vi "unmarshalling.vi"(7 "Type":variant, 8 "error in (no error)":errorcluster, 10 "String":string, 11 "Serializer in":refnum<class "Serializer.JKI-JSON.lvclass">) -> (0 "error out":errorcluster, 2 "Variant":variant, 3 "Serializer out":refnum<class "Serializer.JKI-JSON.lvclass">)   [LabVIEW 2017, in "Serializer.JKI-JSON.lvclass"]
uses:
  Serializer.JKI-JSON.lvclass
  <vilib>/addons/_JKI.lib/Serialization/JSON/JKI JSON Serialization.lvlib
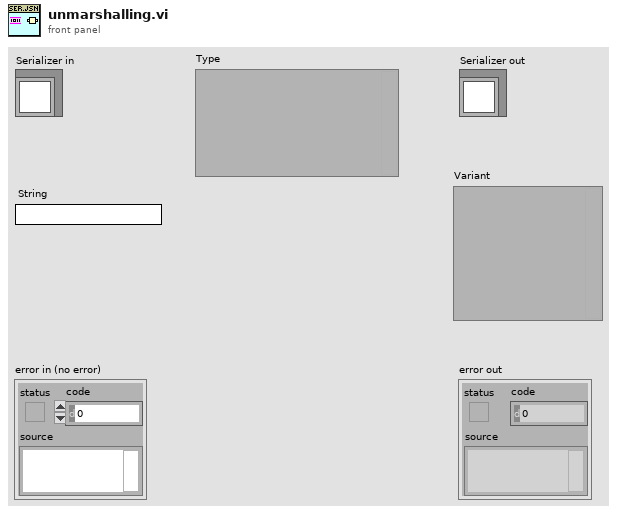
[diagram p1: front panel]
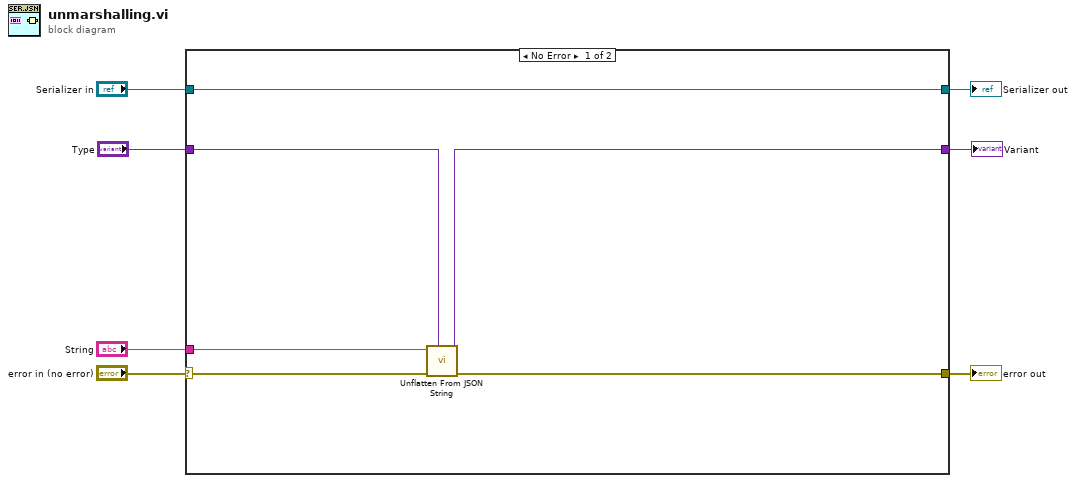
[diagram p0: block diagram]
diagram:
  n1 = case shown="No Error" "error in (no error)" {
    selector: "error in (no error)" -> [w12 w15]
    tunnel: [w8 w15] -> w1
    tunnel: [w13 w14] -> w7
    tunnel: "Serializer in" -> [w13 w14]
    tunnel: [w9 _] -> w6
    tunnel: "Type" -> [w10 _]
    tunnel: "String" -> [w11 _]
    frame No Error {
      n2 = call <vilib>:"Unflatten From JSON String.vi"("Type and Defaults"=w10, "error in (no error)"=w12, "JSON String"=w11) -> ("error out"=w8:errorcluster, "Variant"=w9:variant)  [unwired: 7 in]
    }
    frame Error {
    }
  }
  "error out" <- w1
  "Serializer out" <- w7
  "Variant" <- w6
